vi "相机2拍照.vi"(8 "错误输入（无错误）":errorcluster, 10 "Image":T2, 11 "引用句柄输入":T1) -> (0 "错误输出":errorcluster, 1 "拍照结果":bool, 2 "Image Out":T2, 3 "引用句柄输出":T1)   [LabVIEW 2014]
uses:
  <vilib>/vision/Image Controls.llb/IMAQ Image.ctl
  <vilib>/userdefined/High Color/IMAQdx.ctl
  <vilib>/vision/driver/NI_Vision_Acquisition_Software.lvlib
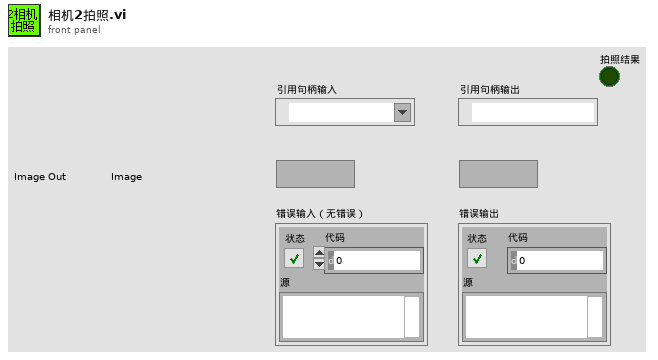
[diagram p1: front panel]
types:
  T1 = typedef "IMAQdx.ctl" = refnum<k21>
  T2 = typedef "IMAQ Image.ctl" = refnum<image>
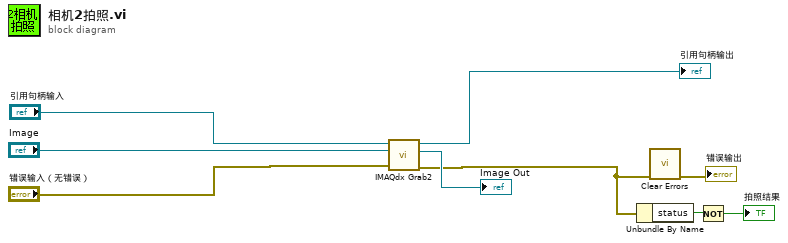
[diagram p0: block diagram]
diagram:
  n1 = call <vilib>:"IMAQdx Grab2.vi"("error in"="错误输入（无错误）", "Image In"="Image", "Session In"="引用句柄输入") -> ("error out"=w3:errorcluster, "Image Out"=→"Image Out":T2, "Session Out"=→"引用句柄输出":T1)  [unwired: 5 in, 1 out]
  n2 = Unbundle By Name(w3) -> ("status"=w2:bool)
  n3 = call <vilib>:"Clear Errors.vi"("error in (no error)"=w3) -> ("error out"=→"错误输出":errorcluster)  [unwired: 5 in, 1 out]
  n4 = Not(x=w2) -> (.not. x?=→"拍照结果":bool)
